vi "FRCts20_Backend_TeamDataSgl.vi"(8 "error in (no error)":errorcluster, 11 "TeamNum":u16) -> (0 "error out":errorcluster, 3 "TeamDataOut":T1)   [LabVIEW 2014, in "FRCts20_Backend_WebMethods.lvlib"]
doc: "The TeamDataSgl function returns to the caller all data describing a single team entry in the overall data set. It accepts a team number as input, and returns a cluster defining the <b>team</b>, <b>number</b>, <b>location</b>, <b>software type</b>, and the <b>issue list</b> for a given team."
uses:
  FRCts20_Backend_WebMethods.lvlib
  FRCts20_Backend_Engine.lvlib
  FRCts20_Backend_FGVOperation.ctl
  FRCts20_Backend_IssueDfn.ctl
  FRCts20_Backend_Controls.lvlib
  FRCts20_Backend_TeamDfn.ctl
  FRCts20_Backend_request_info.ctl
  FRCts20_Backend_Note.ctl
  FRCts20_Backend_Note_list.ctl
  FRCts20_Backend_IssueTeamList.ctl
  FRCts20_Backend_Team_Info.ctl
panel:
  in  "Team":T1
  # "The TeamDataSgl function returns to\nthe caller all data describing a single\nteam entry in the overall data set. It \naccepts a team number as input, and \nreturns a cluster defining the team, \nnumber, location, software type, and \nthe issue list for a given team."
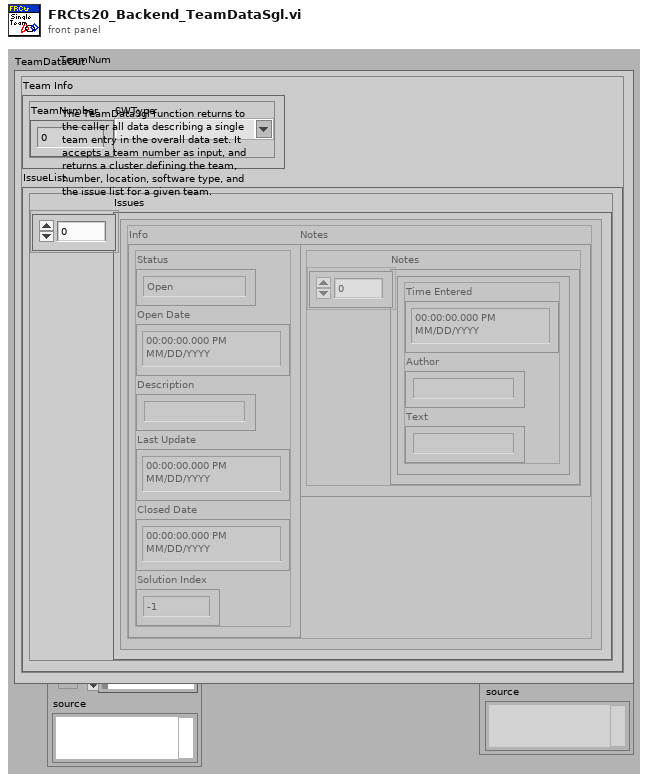
[diagram p1: front panel]
types:
  T1 = typedef "FRCts20_Backend_Controls.lvlib/FRCts20_Backend_TeamDfn.ctl" = cluster{"Team Info":T2, "IssueList":T3}
  T2 = typedef "FRCts20_Backend_Controls.lvlib/FRCts20_Backend_Team_Info.ctl" = cluster{"TeamNumber":u16, "SWType":string}
  T3 = typedef "FRCts20_Backend_Controls.lvlib/FRCts20_Backend_IssueTeamList.ctl" = cluster{"Issues":T4[]}
  T4 = typedef "FRCts20_Backend_Controls.lvlib/FRCts20_Backend_IssueDfn.ctl" = cluster{"Notes":T5, "Info":T7}
  T5 = typedef "FRCts20_Backend_Controls.lvlib/FRCts20_Backend_Note_list.ctl" = cluster{"Notes":T6[]}
  T6 = typedef "FRCts20_Backend_Controls.lvlib/FRCts20_Backend_Note.ctl" = cluster{"Time Entered":timestamp, "Author":string, "Text":string}
  T7 = typedef "FRCts20_Backend_Controls.lvlib/FRCts20_Backend_request_info.ctl" = cluster{"Status":enum16{"Open", "In Work", "Closed"}, "Open Date":timestamp, "Description":string, "Last Update":timestamp, "Closed Date":timestamp, "Solution Index":i32}
  T8 = typedef "FRCts20_Backend_Engine.lvlib/FRCts20_Backend_FGVOperation.ctl" = enum16{"Initialize", "EnqueueMessage", "EnqueueDataReturn", "FlushMessage", "FlushDataReturn"}
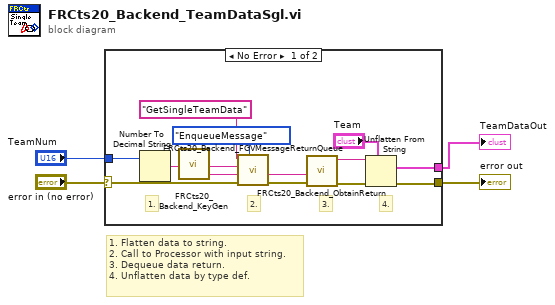
[diagram p0: block diagram]
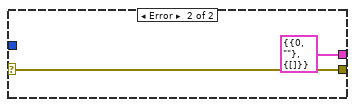
[diagram p2: hidden frame]
diagram:
  # "1. Flatten data to string.\n2. Call to Processor with input string.\n3. Dequeue data return.\n4. Unflatten data by type def."
  n1 = case shown="No Error" "error in (no error)" {
    selector: "error in (no error)" -> [w13 w19]
    tunnel: [w7 w19] -> w3
    tunnel: "TeamNum" -> [w15 _]
    tunnel: [w8 T1 {"Team Info"={"TeamNumber"=0, "SWType"=""}, "IssueList"={"Issues"=[]}} ("Team")] -> w1
    frame No Error {
      # "4."
      # "3."
      # "2."
      # "1."
      n2 = Number To Decimal String(number=w15) -> (decimal integer string=w14:string)  [unwired: 1 in]
      n3 = call "FRCts20_Backend_KeyGen.vi"() -> ("Keygen"=w12:string)  [unwired: 27 in]
      n4 = call "FRCts20_Backend_FGVMessageReturnQueue.vi"("Operation"=FRCts20_Backend_FGVOperation."EnqueueMessage", "error in (no error)"=w13, "Key"=w12, "Message Value"=w14, "Message Name"="GetSingleTeamData") -> ("error out"=w16:errorcluster, "Key (Duplicate)"=w6:string)  [unwired: 3 in]
      n5 = call "FRCts20_Backend_ObtainReturn.vi"("error in (no error)"=w16, "Key"=w6) -> ("error out"=w10:errorcluster, "Message Value"=w5:string)  [unwired: 8 in]
      n6 = Unflatten From String(type="Team", binary string=w5, error in (no error)=w10) -> (value=w8:T1, error out=w7:errorcluster)  [unwired: 2 in, 1 out]
    }
    frame Error {
    }
  }
  "error out" <- w3
  "TeamDataOut" <- w1
